vi "addEdge.vi"(0 "reference":refnum<class "AbstractNode.lvclass">, 1 "egde":refnum<class "AbstractEdge.lvclass">, 2 "p1":T1 {"y" format="%.2f"; "x" format="%.2f"}, 3 "p2":T1 {"y" format="%.2f"; "x" format="%.2f"}, 5 "error in (no error)":errorcluster) -> (14 "reference out":refnum<class "AbstractNode.lvclass">, 15 "edgeHasEndNode":bool, 19 "error out":errorcluster)   [LabVIEW 2012, in "AbstractNode.lvclass"]
doc: "public boolean addEdge(Edge e, Point2D p1, Point2D p2)"
uses:
  <resource>/Framework/Providers/Open_GDS/UML/AbstractNode_class/AbstractNode.lvclass
  <resource>/Framework/Providers/Open_GDS/UML/AbstractEdge_class/AbstractEdge.lvclass
  <resource>/Framework/Providers/Open_GDS/UML/General/Point/Point Point2D.ctl
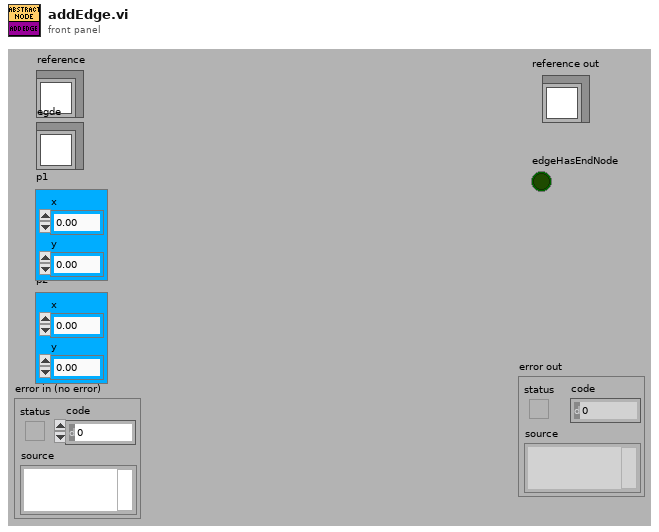
[diagram p1: front panel]
types:
  T1 = typedef "Point Point2D.ctl" = cluster{"x":dbl, "y":dbl}
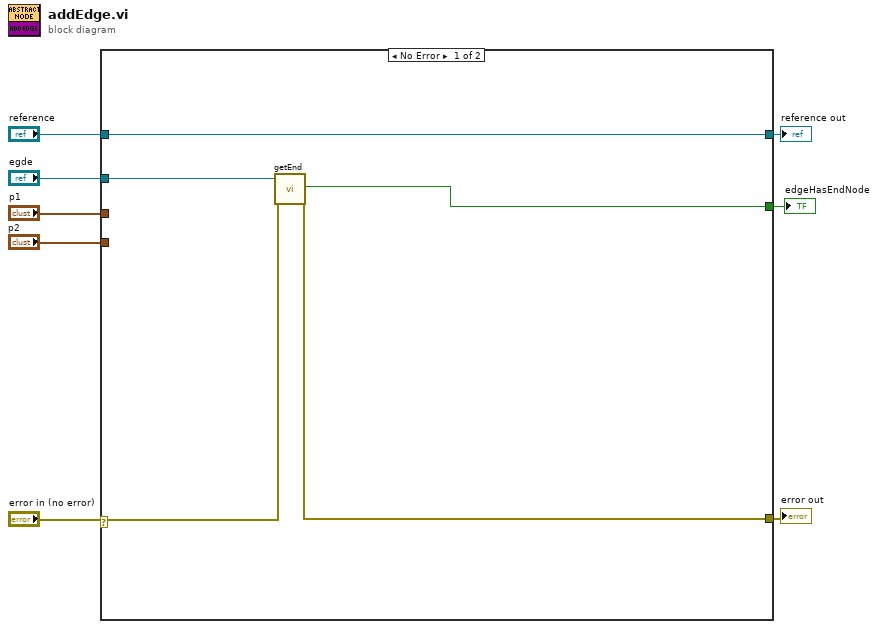
[diagram p0: block diagram]
diagram:
  n1 = case shown="No Error" "error in (no error)" {
    selector: "error in (no error)" -> [w11 w14]
    tunnel: "reference" -> [w13 w15]
    tunnel: [w12 w14] -> w7
    tunnel: [w13 w15] -> w6
    tunnel: "egde" -> [w10 _]
    tunnel: "p1" -> [_ _]
    tunnel: "p2" -> [_ _]
    tunnel: [w9 _] -> w1
    frame No Error {
      n2 = call-dynamic "getEnd.vi"("reference"=w10, "error in (no error)"=w11) -> ("validNode"=w9:bool, "error out"=w12:errorcluster)  [unwired: 14 in, 2 out]
    }
    frame Error {
    }
  }
  "reference out" <- w6
  "error out" <- w7
  "edgeHasEndNode" <- w1
